vi "Project to Plant UML Diagram Script.vi"() -> ()   [LabVIEW 2020]
panel:
  out "DynamicMembers":string[](array[string])
  out "DataMembers":string[](array[string])
  out "StaticMembers":string[](array[string])
  in  "Classes":i32(listbox)=9
  out "Progress:":dbl(slide)=18.0 caption="Complete" scale=0.0..5.0
  in  "Usage":bool=TRUE
  in  "Composition":bool=TRUE
  in  "Inheritance":bool=TRUE
  out "Plant UML Diagram String":string="Alpha_Task_Msg --|> Message\r\nAlpha_Task_Msg --> Alpha\r\nBeta_Task_Msg --|> Message\r\nBeta_Task_Msg --> Beta\r\nLast_Ack --|> Message\r\nLaunch_Nested_Actor_Msg --|> Message\r\nLog_Event_Msg --|> Message\r\nLog_Event_Msg --> Untitled_Project_1\r\nMessage_Priority_Queue --> Message\r\nMessage_Queue --* Message_Priority_Queue\r\nMessage_Queue --> Message\r\nPing_Msg --|> Message\r\nRegister_Actor_Msg --|> Message\r\nStop_Msg --|> Message\r\nUntitled_Project_1 --> Alpha\r\nUntitled_Project_1 --> Beta\r\n"
  in  "Path":path
  # "http://www.plantuml.com/plantuml/uml"
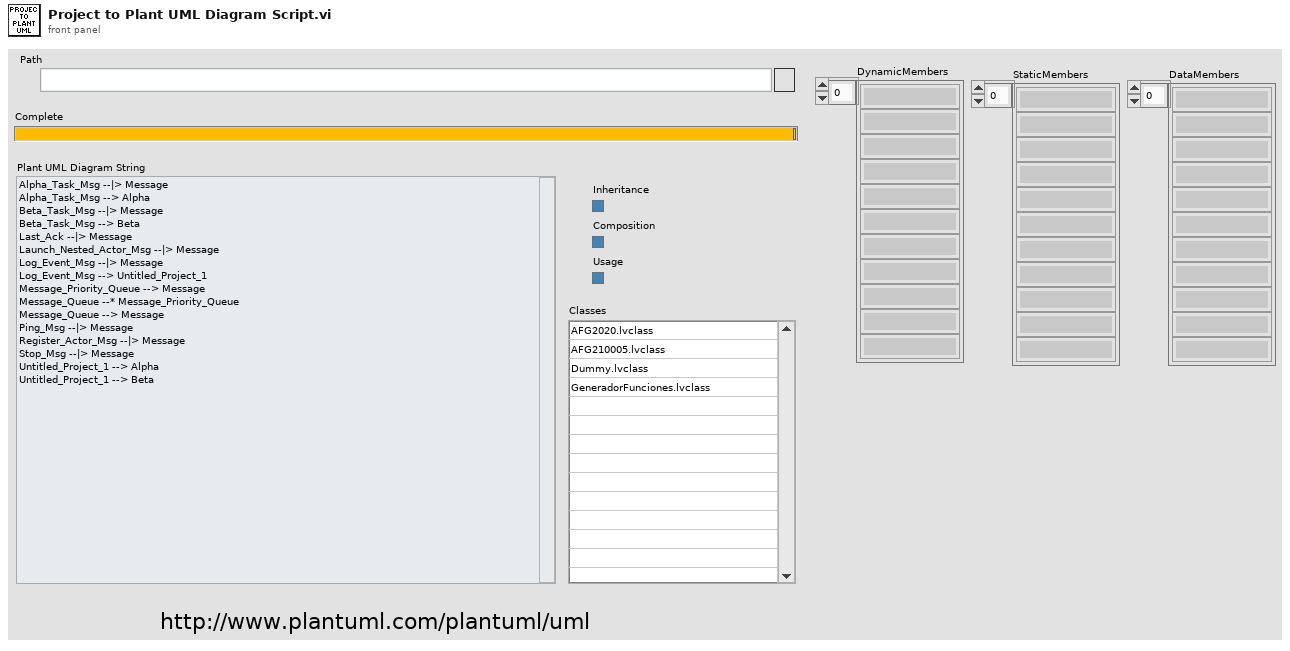
[diagram p1: front panel]
types:
  T1 = cluster{"Class Name":string, "Static Members":string[], "Dynamic Members":string[], "Data Members":string[]}[]
  T2 = map{string, cluster{"Inheritance":set{string}, "Composition":set{string}, "Usage":set{string}}}
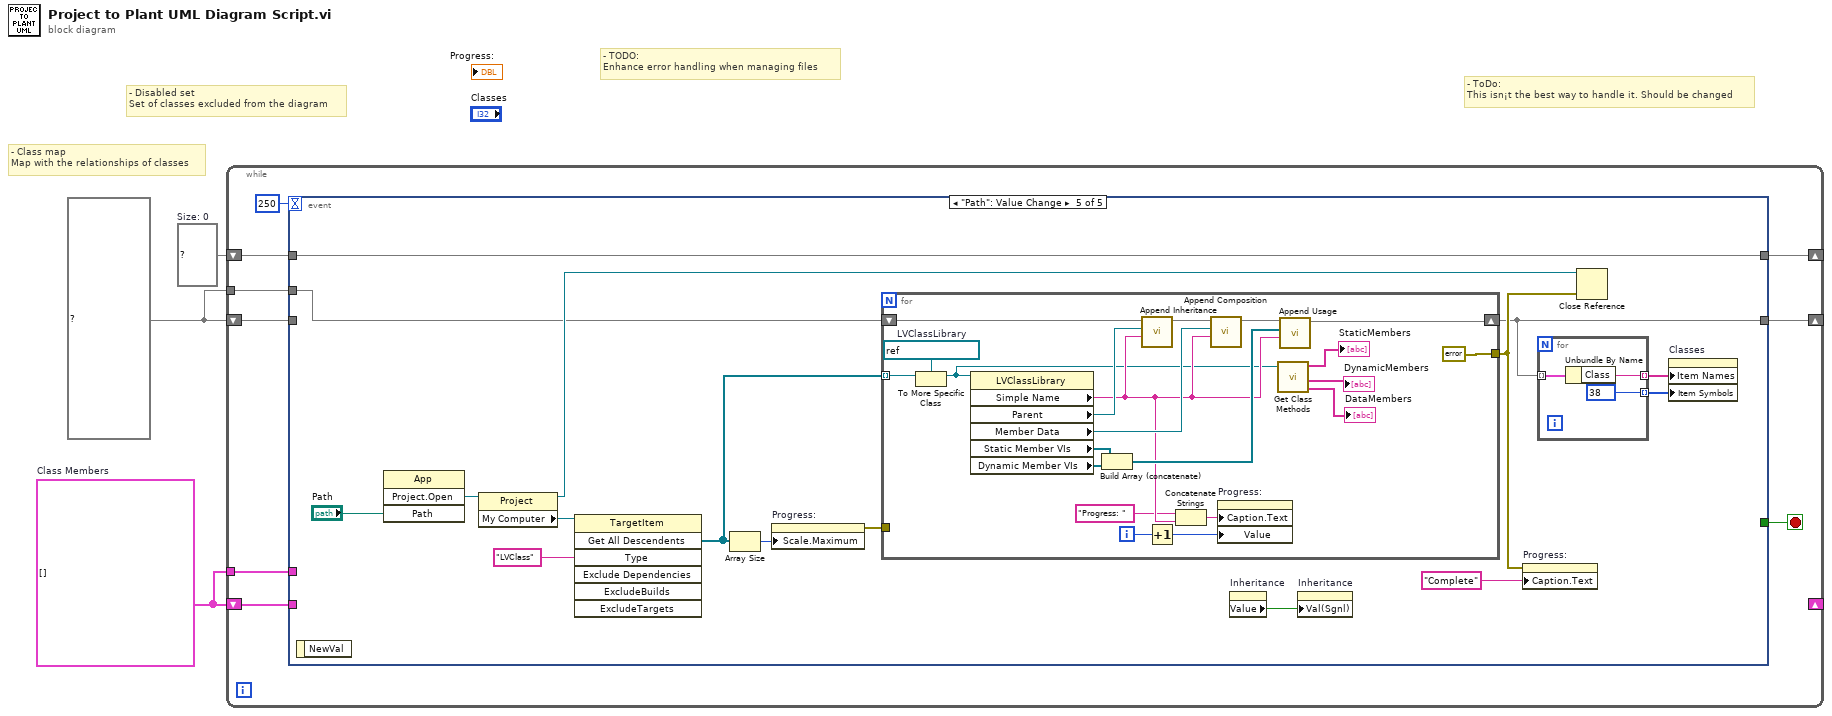
[diagram p0: block diagram]
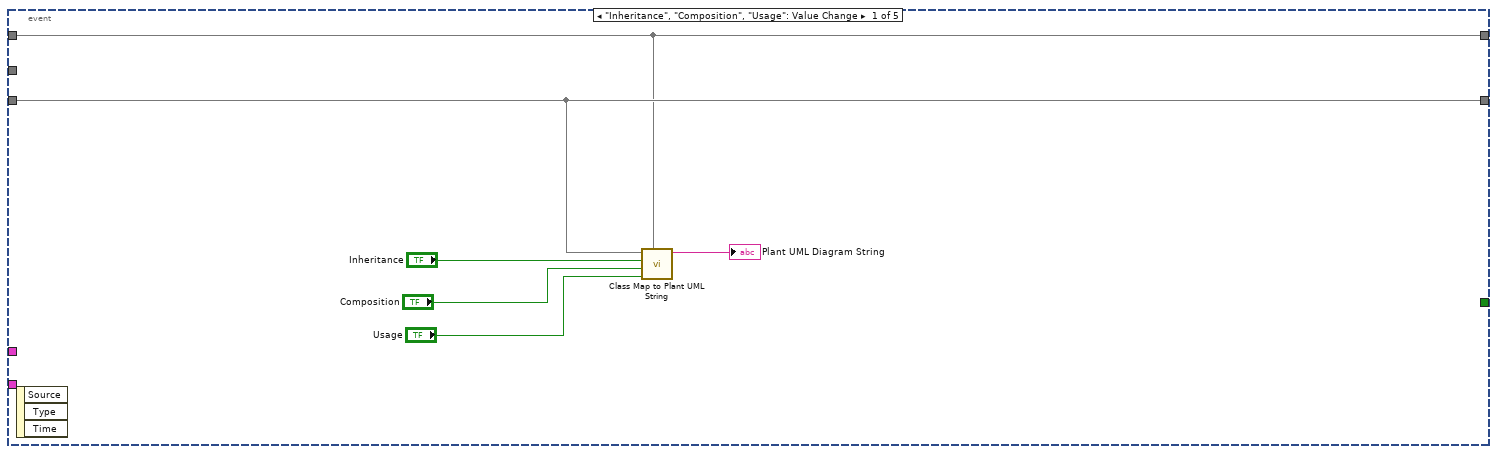
[diagram p2: hidden frame]
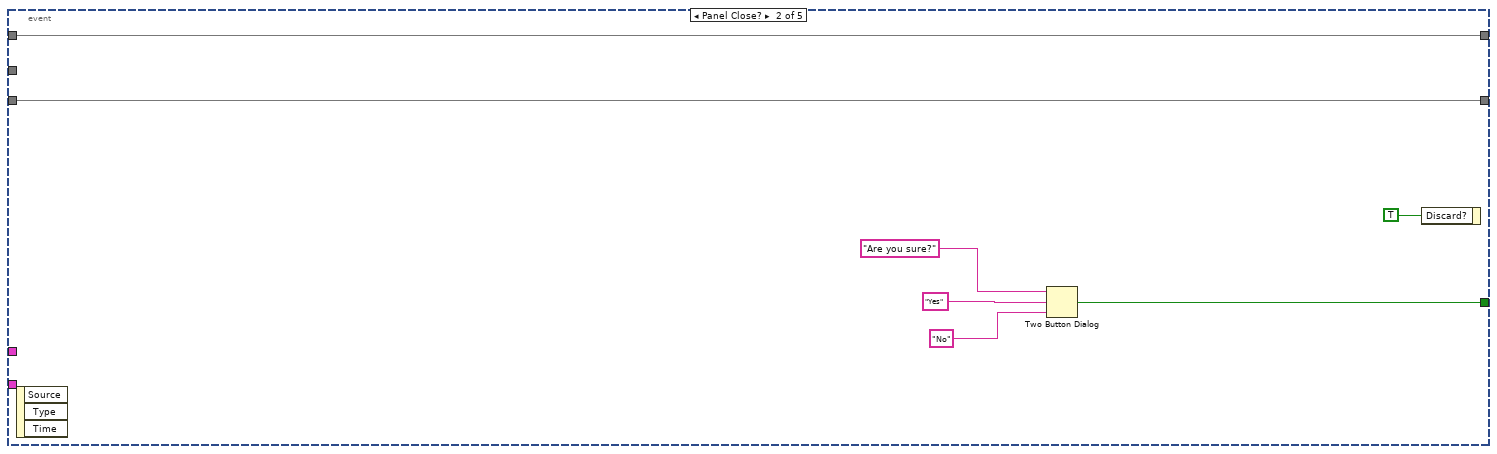
[diagram p3: hidden frame]
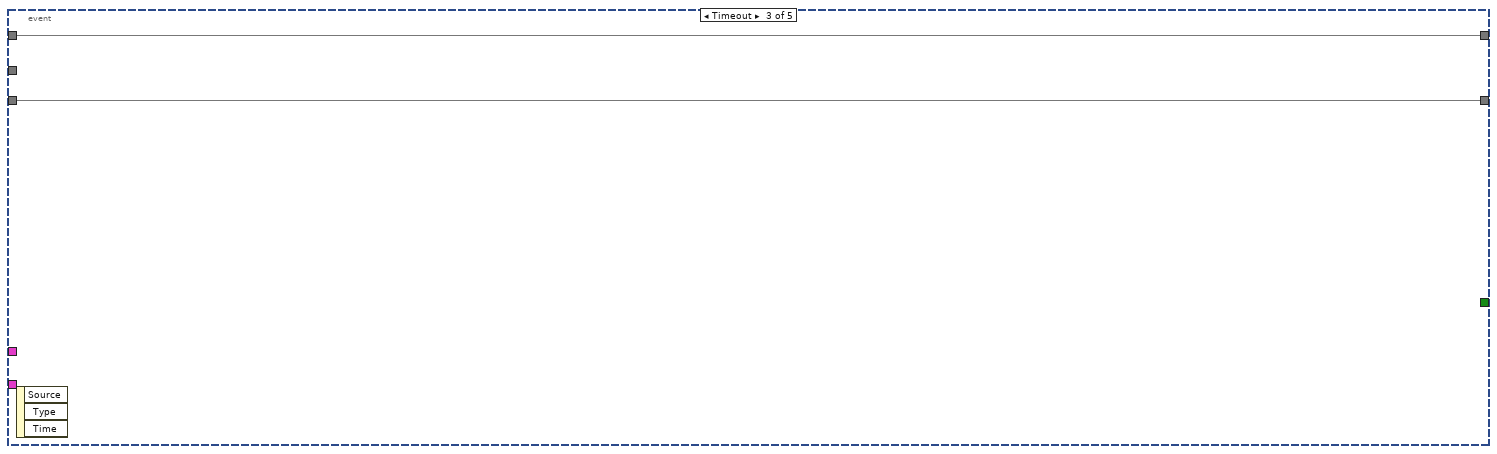
[diagram p4: hidden frame]
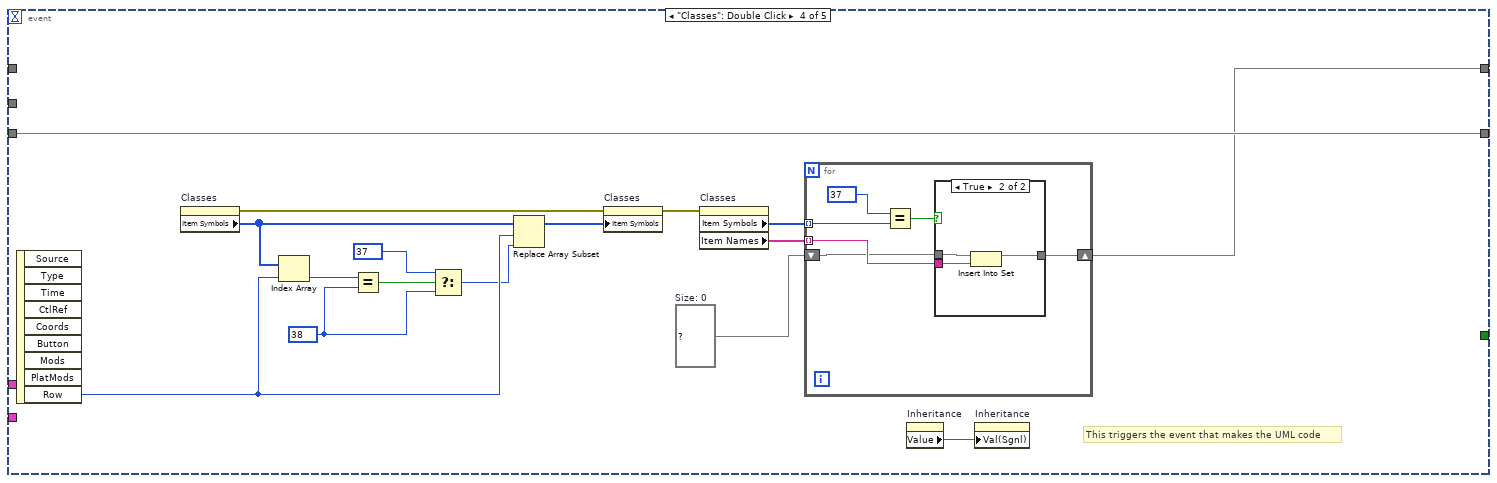
[diagram p5: hidden frame]
diagram:
  w1 = T1 []  # Class Members
  w2 = set{string} {}  # Size: 0
  w3 = T2 {} ("map")
  # "- ToDo:\nThis isn¡t the best way to handle it. Should be changed"
  # "- TODO:\nEnhance error handling when managing files"
  # "- Class map\nMap with the relationships of classes"
  # "- Disabled set\nSet of classes excluded from the diagram"
  n1 = while {
    shift-right: [w10] -> _
    shift-left: w3 -> [w11]
    tunnel: w3 -> [w9]
    shift-right: [w7] -> _
    shift-left: w2 -> [w6]
    tunnel: w1 -> [w4]
    shift-right: _ -> [_]
    shift-left: w1 -> [w5]
    stop <- w8 stop-if-true
    n2 = event shown="[4] \"Path\": Value Change" {
      selector: _ -> [_ _ _ _ _]
      dyn-events: _ -> [_ _ _ _ _]
      timeout: 250 -> [_ _ _ _ _]
      tunnel: w11 -> [w14 w24 w27 w38 _]
      tunnel: [w14 w24 w27 w38 w57] -> w10
      tunnel: w9 -> [_ _ _ _ w62]
      tunnel: [_ w20 _ _ _] -> w8
      tunnel: [w13 w19 w26 w29 w55] -> w7
      tunnel: w6 -> [w13 w19 w26 _ w55]
      tunnel: w5 -> [_ _ _ _ _]
      tunnel: w4 -> [_ _ _ _ _]
      event "Inheritance", "Composition", "Usage": Value Change {
        n3 = event-data() -> ()  [unwired: 1 in, 3 out]
        n4 = call "Class Map to Plant UML String.vi"("Disabled Set"=w13, "Usage"="Usage", "Composition"="Composition", "Inheritance"="Inheritance", "Class Map"=w14) -> ("Plant UML String"=→"Plant UML Diagram String":string)  [unwired: 6 in]
      }
      event Panel Close? {
        n5 = event-data() -> ()  [unwired: 1 in, 3 out]
        n6 = Two Button Dialog(message="Are you sure?", 1:"No" ("F button name (\"Cancel\")"), 2:"Yes" ("T button name (\"OK\")")) -> (T button?=w20:bool)
        n7 = event-data("Discard?"=TRUE) -> ()  [unwired: 1 in, 1 out]
      }
      event Timeout {
        n8 = event-data() -> ()  [unwired: 1 in, 3 out]
      }
      event "Classes": Double Click {
        w30 = set{string} {}  # Size: 0
        w40 = 38
        # "This triggers the event that makes the UML code"
        n9 = event-data() -> ("Row"=w36:i32)  [unwired: 1 in, 8 out]
        n10 = property on="Classes" class="LstBox (strict)"() -> (error out=w39:errorcluster, "Item Symbols"=w37:i32[])  [unwired: 2 in, 1 out]
        n11 = Index Array(array=w37, index=w36) -> (element=w43:i32)
        n12 = Equal?(x=w43, y=w40) -> (x = y?=w42:bool)
        n13 = Select(t=37, s=w42, f=w40) -> (s? t:f=w35:i32)
        n14 = Replace Array Subset(array=w37, new element=w35, index=w36) -> (w34:i32[])
        n15 = property on="Classes" class="LstBox (strict)"(error in=w39, "Item Symbols"=w34) -> (error out=w33:errorcluster)  [unwired: 1 in, 1 out]
        n16 = property on="Classes" class="LstBox (strict)"(error in=w33) -> ("Item Symbols"=w32:i32[], "Item Names"=w31:string[])  [unwired: 1 in, 2 out]
        n17 = for {
          tunnel: w32 -> [w49] mode=indexing
          tunnel: w31 -> [w46] mode=indexing
          shift-right: [w45] -> w29
          shift-left: w30 -> [w44]
          n18 = Equal?(x=37, y=w49) -> (x = y?=w47:bool)
          n19 = case shown="True" w47 {
            tunnel: w46 -> [_ w53]
            tunnel: [w50 w52] -> w45
            tunnel: w44 -> [w50 w51]
            frame False {
            }
            frame True {
              n20 = Insert Into Set(10:w53, 11:w51) -> (3:w52:set{string})  [unwired: 1 out]
            }
          }
        }
        n21 = property on="Inheritance" class="Bool (strict)"() -> ("Value"=w28:bool)  [unwired: 2 in, 2 out]
        n22 = property on="Inheritance" class="Bool (strict)"("Val(Sgnl)"=w28) -> ()  [unwired: 2 in, 2 out]
      }
      event "Path": Value Change {
        n23 = event-data() -> ()  [unwired: 1 in, 1 out]
        n24 = invoke class="App" method="Project.Open"("Path"="Path") -> ("Project:Open"=w68:refnum<vi>)  [unwired: 3 in, 3 out]
        n25 = property class="Project"(reference=w68) -> (reference out=w63:refnum<vi>, "My Computer"=w69:refnum<vi>)  [unwired: 1 in, 1 out]
        n26 = invoke class="TargetItem" method="Get All Descendents"(reference=w69, "Type"="LVClass") -> ("All Descendents"=w64:refnum<vi>[])  [unwired: 5 in, 6 out]
        n27 = Array Size(array=w64) -> (size(s)=w60:i32)
        n28 = property on="Progress:" class="Slide (strict)"("Scale.Maximum"=w60) -> (error out=w65:errorcluster)  [unwired: 2 in, 1 out]
        n29 = for {
          tunnel: w64 -> [w93] mode=indexing
          shift-right: [w84] -> w57
          shift-left: w62 -> [w87]
          tunnel: [errorcluster {"status"=FALSE, "code"=0, "source"=""} ("error constant")] -> w59
          tunnel: w65 -> [_]
          i -> [w80]
          w92 = refnum<vi> refnum  # LVClassLibrary
          n30 = To More Specific Class(target class=w92, reference=w93) -> (specific class reference=w76:refnum<vi>)  [unwired: 1 in, 1 out]
          n31 = property class="LVClassLibrary"(reference=w76) -> ("Simple Name"=w82:string, "Parent"=w86:refnum<vi>, "Member Data"=w88:refnum<vi>, "Static Member VIs"=w91:refnum<vi>[], "Dynamic Member VIs"=w90:refnum<vi>[])  [unwired: 1 in, 2 out]
          n32 = Build Array (concatenate)(w91, w90) -> (w89:refnum<vi>[])
          n33 = call "Append Inheritance.vi"("Class"=w82, "Parent Class"=w86, "Class Relations Map"=w87) -> ("Class Relations Map Out"=w78:T2)  [unwired: 8 in]
          n34 = Increment(x=w80) -> (x+1=w77:i32)
          n35 = Concatenate Strings("Progress: " ("string"), w82) -> (w83:string)
          n36 = call "Append Composition.vi"("Class"=w82, "Private Data Control"=w88, "Class Relations Map"=w78) -> ("Class Relations Map Out"=w79:T2)  [unwired: 8 in]
          n37 = property on="Progress:" class="Slide (strict)"("Caption.Text"=w83, "Value"=w77) -> ()  [unwired: 2 in, 2 out]
          n38 = call "Get Class Methods.vi"("LVClassLibrary Refnum"=w76) -> ("DataMembers"=→"DataMembers":string[], "DynamicMembers"=→"DynamicMembers":string[], "StaticMembers"=→"StaticMembers":string[])  [unwired: 6 in]
          n39 = call "Append Usage.vi"("Class"=w82, "VIs"=w89, "Class Relations Map"=w79) -> ("Class Relations Map Out"=w84:T2)  [unwired: 8 in]
        }
        n40 = property on="Inheritance" class="Bool (strict)"() -> ("Value"=w54:bool)  [unwired: 2 in, 2 out]
        n41 = property on="Inheritance" class="Bool (strict)"("Val(Sgnl)"=w54) -> ()  [unwired: 2 in, 2 out]
        n42 = property on="Progress:" class="Slide (strict)"(error in=w59, "Caption.Text"="Complete") -> ()  [unwired: 1 in, 2 out]
        n43 = for {
          tunnel: [w71] -> w58 mode=indexing
          tunnel: w57 -> [w72] mode=indexing
          tunnel: [38] -> w56 mode=indexing
          n44 = Unbundle By Name(w72) -> ("Class"=w71:string)
        }
        n45 = Close Reference(reference=w63, error in (no error)=w59) -> ()  [unwired: 1 out]
        n46 = property on="Classes" class="LstBox (strict)"("Item Names"=w58, "Item Symbols"=w56) -> ()  [unwired: 2 in, 2 out]
      }
    }
  }
